vi "GetChangedEdges.vi"(8 "error in (no error)":errorcluster, 10 "Apply Updates (F)":bool, 11 "DirectedGraphWorldMap in":refnum<class "NI_Robotics_DirectedGraphWorldMap.lvclass">) -> (0 "error out":errorcluster, 2 "Changed Edges":T1[](array[typedef]), 3 "DirectedGraphWorldMap out":refnum<class "NI_Robotics_DirectedGraphWorldMap.lvclass">)   [LabVIEW 2017, in "NI_Robotics_DirectedGraphWorldMap.lvclass"]
uses:
  <vilib>/robotics/Navigation/shared/WorldMap/DirectedGraphWorldMap/NI_Robotics_DirectedGraphWorldMap.lvclass
  <vilib>/robotics/Navigation/shared/WorldMap/World Map Edge.ctl
  <vilib>/robotics/Navigation/shared/MapNode/AbstractMapNode/NI_Robotics_AbstractMapNode.lvclass
  <vilib>/robotics/Navigation/shared/WorldMap/DirectedGraphWorldMap/NI_Robotics_DirectedGraphWorldMap.lvclass/NI_Robotics_DirectedGraphWorldMap.ctl
  <vilib>/robotics/Navigation/shared/MapNode/DirectedGraphMapNode/NI_Robotics_DirectedGraphMapNode.lvclass
  c:/Program Files (x86)/National Instruments/LabVIEW 2017/vi.lib/robotics/Navigation/shared/MapNode/AbstractMapNode/NI_Robotics_AbstractMapNode.lvclass
  <vilib>/robotics/Navigation/shared/WorldMap/AbstractWorldMap/NI_Robotics_AbstractWorldMap.lvclass
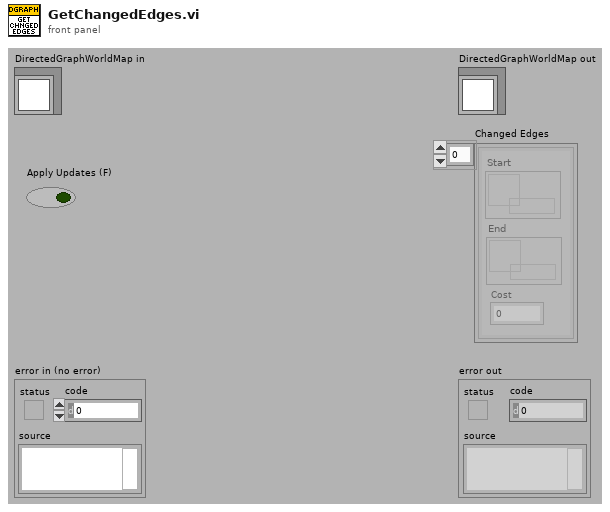
[diagram p1: front panel]
types:
  T1 = typedef "NI_Robotics_AbstractWorldMap.lvclass/World Map Edge.ctl" = cluster{"Start":refnum<data-value>, "End":refnum<data-value>, "Cost":dbl}
  T2 = cluster{"Start":string, "End":string, "Cost":dbl}[]
  T3 = cluster{"Node ref":refnum<data-value>, "Node ref":refnum<data-value>, "Cost":dbl}
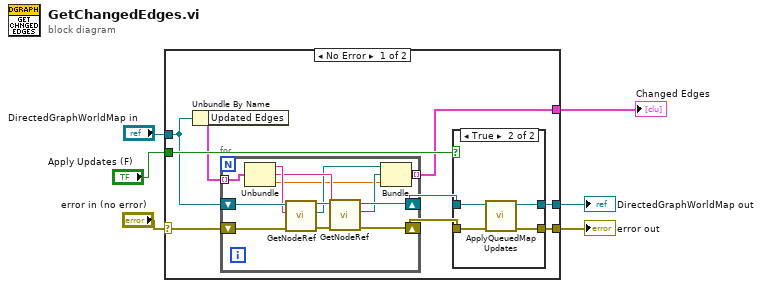
[diagram p0: block diagram]
diagram:
  n1 = case shown="No Error" "error in (no error)" {
    selector: "error in (no error)" -> [w12 w36]
    tunnel: [w13 w36] -> w5
    tunnel: "Apply Updates (F)" -> [w15 _]
    tunnel: "DirectedGraphWorldMap in" -> [w11 w35]
    tunnel: [w7 _] -> w2
    tunnel: [w14 w35] -> w1
    frame No Error {
      n2 = Unbundle By Name(w11) -> ("Updated Edges"=w8:T2)
      n3 = for {
        shift-right: [w25] -> w10
        shift-left: w11 -> [w27]
        shift-right: [w23] -> w9
        shift-left: w12 -> [w28]
        tunnel: w8 -> [w22] mode=indexing
        tunnel: [w16] -> w7 mode=indexing
        n4 = Unbundle(w22) -> ("Start"=w21:string, "End"=w20:string, "Cost"=w17:dbl)
        n5 = call <vilib>:"GetNodeRef.vi"("error in (no error)"=w28, "Node Name"=w21, "DirectedGraphWorldMap in"=w27) -> ("error out"=w24:errorcluster, "Node ref"=w19:refnum<data-value>, "DirectedGraphWorldMap out"=w26:refnum<class "NI_Robotics_DirectedGraphWorldMap.lvclass">)  [unwired: 5 in, 1 out]
        n6 = call <vilib>:"GetNodeRef.vi"("error in (no error)"=w24, "Node Name"=w20, "DirectedGraphWorldMap in"=w26) -> ("error out"=w23:errorcluster, "Node ref"=w18:refnum<data-value>, "DirectedGraphWorldMap out"=w25:refnum<class "NI_Robotics_DirectedGraphWorldMap.lvclass">)  [unwired: 5 in, 1 out]
        n7 = Bundle("Node ref"=w19, "Node ref"=w18, "Cost"=w17) -> (w16:T3)  [unwired: 1 in]
      }
      n8 = case shown="True" w15 {
        tunnel: w10 -> [w30 w34]
        tunnel: [w30 w32] -> w14
        tunnel: w9 -> [w29 w33]
        tunnel: [w29 w31] -> w13
        frame False {
        }
        frame True {
          n9 = call-dynamic "ApplyQueuedMapUpdates.vi"("error in (no error)"=w33, "DirectedGraphWorldMap in"=w34) -> ("error out"=w31:errorcluster, "DirectedGraphWorldMap out"=w32:refnum<class "NI_Robotics_DirectedGraphWorldMap.lvclass">)  [unwired: 8 in]
        }
      }
    }
    frame Error {
    }
  }
  "error out" <- w5
  "DirectedGraphWorldMap out" <- w1
  "Changed Edges" <- w2
